vi "LED_rand_wait.vi"(5 "FPGA I/O In":refnum<k21>="IO Module\\D0 0", 6 "Randomly generated testpulse separation input (20 ns ticks)":u32=50000, 7 "Testpulser On/Off":bool, 10 "Testpulse Time Delay (20 ns ticks)":u32=15, 11 "Testpulse duration (20 ns ticks)":u32=1) -> (1 "Is Test Pulse?":bool, 3 "Get New Value":bool)   [LabVIEW 2012]
uses:
  <vilib>/eio/EIONode/EIONode.xnode
  <vilib>/rvi/eio/common/nirviEmuTemplateMethod_errors.vi
panel:
  out "Separation distance counter":u32
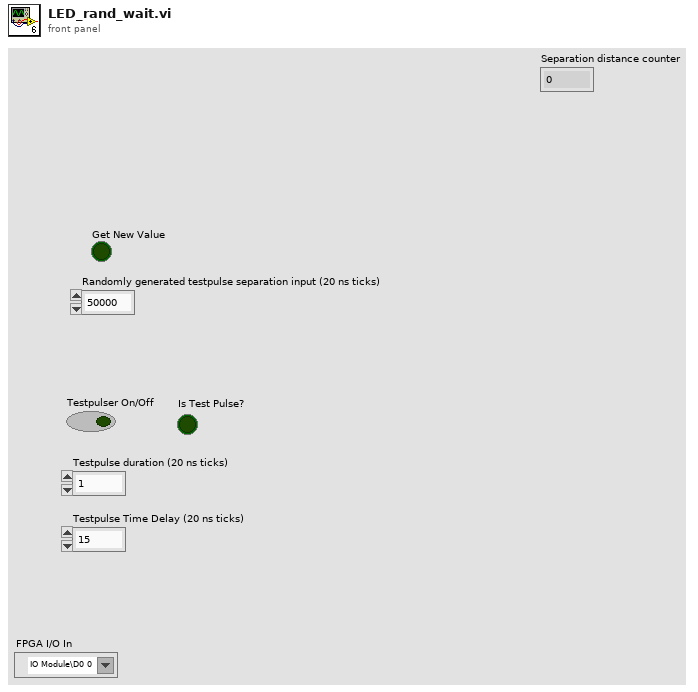
[diagram p1: front panel]
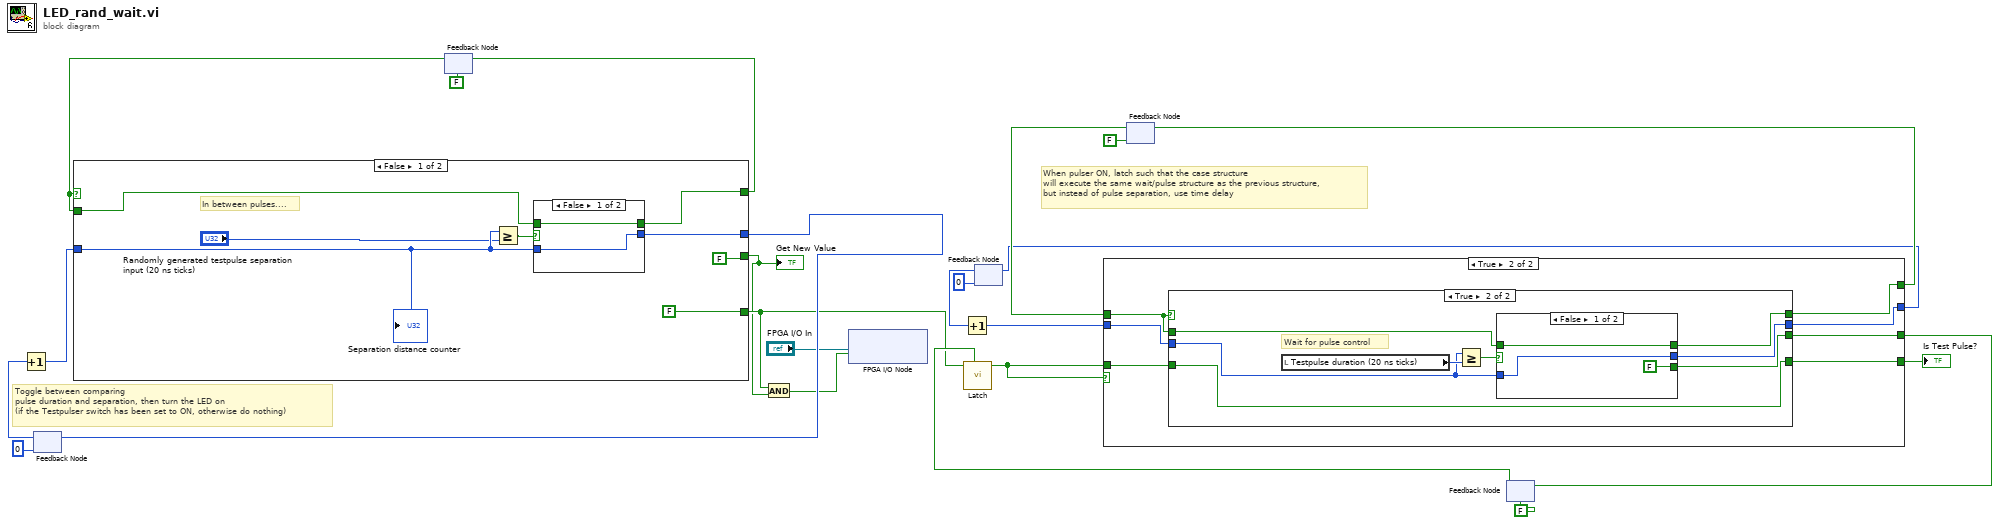
[diagram p0: block diagram]
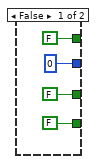
[diagram p2: hidden frame]
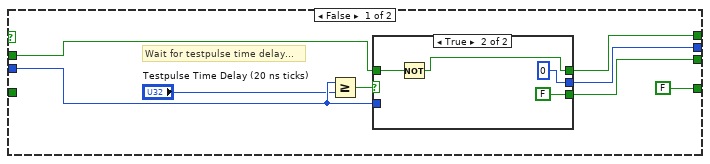
[diagram p3: hidden frame]
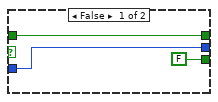
[diagram p4: hidden frame]
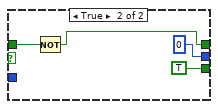
[diagram p5: hidden frame]
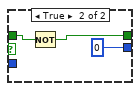
[diagram p6: hidden frame]
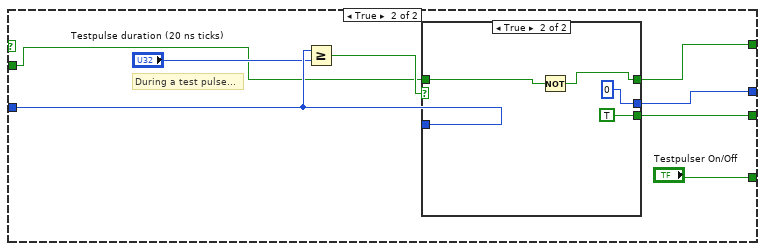
[diagram p7: hidden frame]
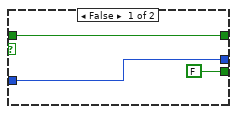
[diagram p8: hidden frame]
diagram:
  # "Toggle between comparing \npulse duration and separation, then turn the LED on\n(if the Testpulser switch has been set to ON, otherwise do nothing)"
  # "When pulser ON, latch such that the case structure\nwill execute the same wait/pulse structure as the previous structure, \nbut instead of pulse separation, use time delay"
  n1 = feedback #1(u32 0) -> (w8:u32)
  n2 = Increment(x=w8) -> (x+1=w5:u32)
  n3 = feedback #2(FALSE) -> (w11:bool)
  n4 = case shown="False" w11 {
    tunnel: w5 -> [w28 w41]
    tunnel: [w31 w43] -> w9
    tunnel: [w30 w44] -> w19
    tunnel: [FALSE ("IO Module\\D0 0") "Testpulser On/Off"] -> w3
    tunnel: w11 -> [w26 w38]
    tunnel: [FALSE w37] -> w1
    frame False {
      # "In between pulses...."
      n5 = Greater Or Equal?(x=w28, y="Randomly generated testpulse separation input (20 ns ticks)") -> (x >= y?=w27:bool)
      n6 = case shown="False" w27 {
        tunnel: [w33 u32 0] -> w31
        tunnel: w28 -> [w33 _]
        tunnel: [w32 w35] -> w30
        tunnel: w26 -> [w32 w34]
        frame False {
        }
        frame True {
          n7 = Not(x=w34) -> (.not. x?=w35:bool)
        }
      }
      "Separation distance counter" <- w28
    }
    frame True {
      # "During a test pulse..."
      n8 = Greater Or Equal?(x=w41, y="Testpulse duration (20 ns ticks)") -> (x >= y?=w40:bool)
      n9 = case shown="True" w40 {
        tunnel: w41 -> [w47 _]
        tunnel: [w46 w51] -> w44
        tunnel: [w47 u32 0] -> w43
        tunnel: w38 -> [w46 w49]
        tunnel: [FALSE TRUE] -> w37
        frame False {
        }
        frame True {
          n10 = Not(x=w49) -> (.not. x?=w51:bool)
        }
      }
    }
  }
  "Get New Value" <- w1
  n11 = feedback-in #1(w9) -> ()
  n12 = feedback-in #2(w19) -> ()
  n13 = And(x=w3, y=w1) -> (x .and. y?=w2:bool)
  n14 = xnode "FPGA I/O Node"("I/O Item"=w2, "FPGA I/O In"="FPGA I/O In") -> ()  [unwired: 1 out]
  n15 = feedback #3(u32 0) -> (w13:u32)
  n16 = Increment(x=w13) -> (x+1=w14:u32)
  n17 = feedback #4(FALSE) -> (w17:bool)
  n18 = feedback #5(FALSE) -> (w22:bool)
  n19 = call "Latch.vi"("Reset"=w22, "Input"=w3) -> ("Output"=w23:bool)  [unwired: 9 in]
  n20 = case shown="True" w23 {
    tunnel: w23 -> [_ w57]
    tunnel: [FALSE w59] -> w6
    tunnel: w14 -> [_ w60]
    tunnel: [u32 0 w58] -> w15
    tunnel: w17 -> [_ w62]
    tunnel: [FALSE w61] -> w18
    tunnel: [FALSE w56] -> w21
    frame False {
    }
    frame True {
      n21 = case shown="True" w62 {
        tunnel: w62 -> [w69 w82]
        tunnel: [w68 w81] -> w61
        tunnel: w60 -> [w65 w83]
        tunnel: [FALSE w79] -> w59
        tunnel: [w66 w80] -> w58
        tunnel: w57 -> [_ w79]
        tunnel: [w63 w78] -> w56
        frame False {
          # "Wait for testpulse time delay..."
          n22 = Greater Or Equal?(x=w65, y="Testpulse Time Delay (20 ns ticks)") -> (x >= y?=w70:bool)
          n23 = case shown="True" w70 {
            tunnel: w69 -> [w73 w77]
            tunnel: [w73 w76] -> w68
            tunnel: [w72 u32 0] -> w66
            tunnel: w65 -> [w72 _]
            tunnel: [FALSE FALSE] -> w63
            frame False {
            }
            frame True {
              n24 = Not(x=w77) -> (.not. x?=w76:bool)
            }
          }
        }
        frame True {
          # "Wait for pulse control"
          n25 = local read "Testpulse duration (20 ns ticks)"() -> (w85:u32)
          n26 = Greater Or Equal?(x=w83, y=w85) -> (x >= y?=w84:bool)
          n27 = case shown="False" w84 {
            tunnel: w83 -> [w87 _]
            tunnel: w82 -> [w88 w91]
            tunnel: [w88 w90] -> w81
            tunnel: [w87 u32 0] -> w80
            tunnel: [FALSE TRUE] -> w78
            frame False {
            }
            frame True {
              n28 = Not(x=w91) -> (.not. x?=w90:bool)
            }
          }
        }
      }
    }
  }
  "Is Test Pulse?" <- w6
  n29 = feedback-in #3(w15) -> ()
  n30 = feedback-in #4(w18) -> ()
  n31 = feedback-in #5(w21) -> ()
